vi "get sampling info.vi"(8 "error in (no error)":errorcluster, 11 "ImagingModeSPIM in":refnum<class "ImagingModeSPIM.lvclass">) -> (0 "error out":errorcluster, 3 "ImagingModeSPIM out":refnum<class "ImagingModeSPIM.lvclass">)   [LabVIEW 2012, in "ImagingModeSPIM.lvclass"]
uses:
  ImagingModeSPIM.lvclass
  ImagingModeSPIM.lvclass/ImagingModeSPIM.ctl
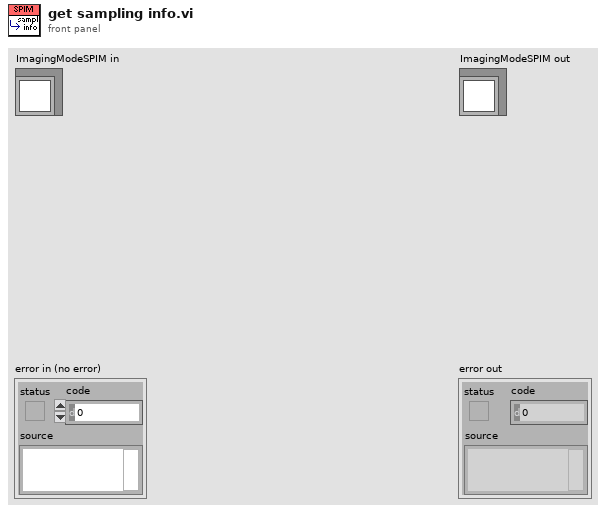
[diagram p1: front panel]
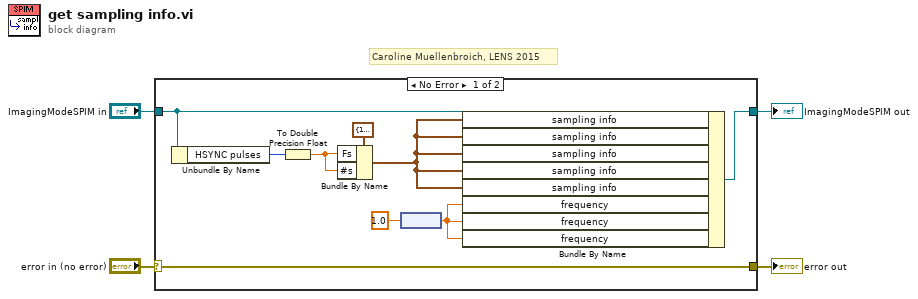
[diagram p0: block diagram]
diagram:
  # "Caroline Muellenbroich, LENS 2015"
  n1 = case shown="No Error" "error in (no error)" {
    selector: "error in (no error)" -> [w13 w15]
    tunnel: [w13 w15] -> w3
    tunnel: [w10 w14] -> w1
    tunnel: "ImagingModeSPIM in" -> [w11 w14]
    frame No Error {
      n2 = Unbundle By Name(w11) -> ("HSYNC pulses"=w12:i32)
      n3 = To Double Precision Float(number=w12) -> (double precision float=w8:dbl)
      n4 = Bundle By Name(cluster=cluster{"Fs":dbl, "#s":dbl} {"Fs"=1000.0, "#s"=1000.0} ("sampling info 2"), "Fs"=w8, "#s"=w8) -> (w5:cluster{"Fs":dbl, "#s":dbl})
      n5 = node(1.0) -> (w6:dbl[unit])
      n6 = Bundle By Name(cluster=w11, "sampling info"=w5, "sampling info"=w5, "sampling info"=w5, "sampling info"=w5, "sampling info"=w5, "frequency"=w6, "frequency"=w6, "frequency"=w6) -> (w10:refnum<class "ImagingModeSPIM.lvclass">)
    }
    frame Error {
    }
  }
  "error out" <- w3
  "ImagingModeSPIM out" <- w1
